vi "Run.vi"(8 "error in (no error)":errorcluster, 11 "Save Image in":refnum<class "Save Image.lvclass">) -> (0 "error out":errorcluster, 3 "Save Image out":refnum<class "Save Image.lvclass">)   [LabVIEW 2018, in "Save Image.lvclass"]
uses:
  Save Image.lvclass
  Save Image.lvclass/Save Image.ctl
  State Machine/State Machine.lvclass
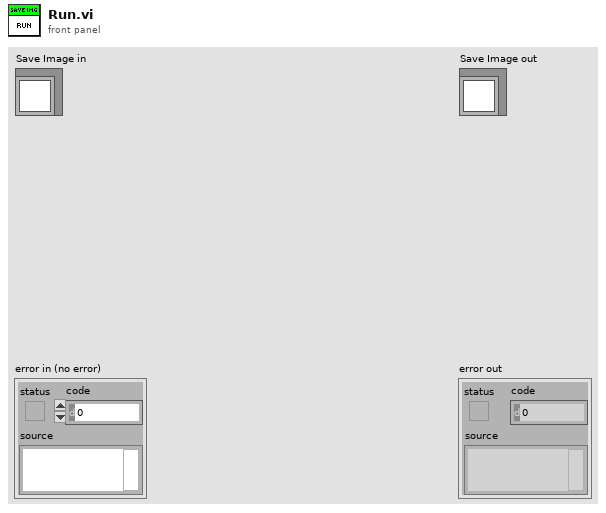
[diagram p1: front panel]
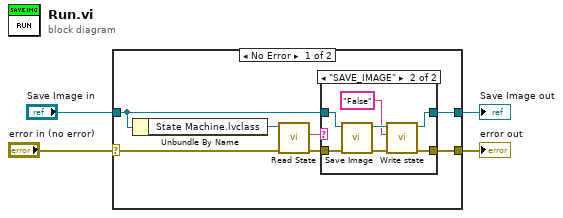
[diagram p0: block diagram]
diagram:
  n1 = case shown="No Error" "error in (no error)" {
    selector: "error in (no error)" -> [w10 w22]
    tunnel: [w5 w22] -> w3
    tunnel: [w6 w21] -> w2
    tunnel: "Save Image in" -> [w8 w21]
    frame No Error {
      n2 = Unbundle By Name(w8) -> ("State Machine.lvclass"=w11:refnum<class "State Machine.lvclass">)
      n3 = call-dynamic "Read State.vi"("error in (no error)"=w10, "State Machine in"=w11) -> ("error out"=w7:errorcluster, "State"=w9:string)  [unwired: 7 in, 1 out]
      n4 = case shown="\"SAVE_IMAGE\"" w9 {
        tunnel: w8 -> [w13 w20]
        tunnel: w7 -> [w12 w19]
        tunnel: [w13 w18] -> w6
        tunnel: [w12 w17] -> w5
        frame "False", Default {
        }
        frame "SAVE_IMAGE" {
          n5 = call "Save Image.vi"("error in (no error)"=w19, "Save Image in"=w20) -> ("error out"=w16:errorcluster, "Save Image out"=w15:refnum<class "Save Image.lvclass">)  [unwired: 8 in]
          n6 = call "Write state.vi"("error in (no error)"=w16, "String"="False", "Save Image in"=w15) -> ("error out"=w17:errorcluster, "Save Image out"=w18:refnum<class "Save Image.lvclass">)  [unwired: 7 in]
        }
      }
    }
    frame Error {
    }
  }
  "error out" <- w3
  "Save Image out" <- w2
